vi "FGV_PROXY_connection_references.vi"(6 "station":T1, 7 "options":T2, 8 "error_in":errorcluster, 11 "reference_in":refnum<k5>) -> (0 "error_out":errorcluster, 1 "killed?":bool, 2 "connection_ID_out":refnum<k5>, 3 "listener_ID_out":refnum<k5>)   [LabVIEW 2020]
uses:
  FGV_PROXY_connection_references.ctl
  STATION/station.ctl
  main_ini/FGV_PROXY_config_info.ctl
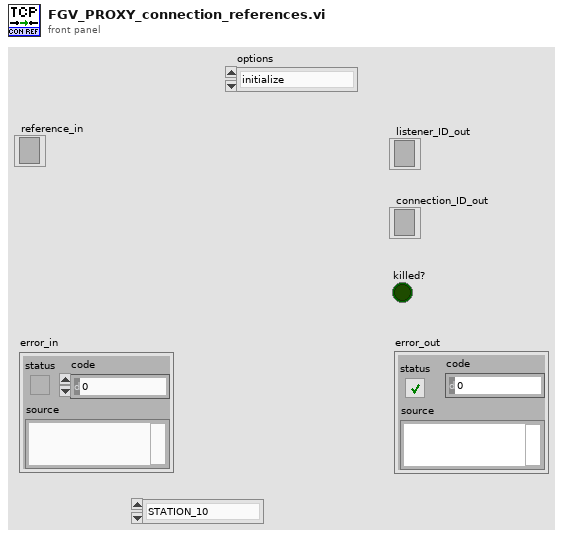
[diagram p1: front panel]
types:
  T1 = typedef "station.ctl" = enum16{"STATION_10", "STATION_20", "STATION_30", "STATION_40", "STATION_50", "STATION_60", "STATION_70", "STATION_80", "STATION_90", "STATION_100", "STATION_110", "STATION_120", "STATION_165", "MAIN"}
  T2 = typedef "FGV_PROXY_connection_references.ctl" = enum16{"initialize", "set_listener_ID", "set_connection_ID", "get", "KILL_ALL_CONNECTIONS", "killed?"}
  T3 = typedef "FGV_PROXY_config_info.ctl" = enum16{"initialize", "set", "get"}
  T4 = typedef "PROXY_all_config_info.ctl" = cluster{"main_ini_file":T5, "SQL Password":string, "queue_refnums":T6, "number_of_stations":i32}
  T5 = typedef "PROXY_main_ini_file.ctl" = cluster{"SQL Driver":string, "SQL Server":string, "SQL Database":string, "SQL UID":string, "Reference table":string, "Reference history":string, "Archivisation CFG table":string, "Archivisation CFG history":string, "User table":string, "User history":string, "default language":string, "REF CHG listener IP":string, "REF CHG listener port":u16, "ST 10 name":string, "ST 10 listener IP":string, "ST 10 listener port":u16, "ST 20 name":string, "ST 20 listener IP":string, "ST 20 listener port":u16, "ST 30 name":string, "ST 30 listener IP":string, "ST 30 listener port":u16, "ST 40 name":string, "ST 40 listener IP":string, "ST 40 listener port":u16, "ST 50 name":string, "ST 50 listener IP":string, "ST 50 listener port":u16, "ST 60 name":string, "ST 60 listener IP":string, "ST 60 listener port":u16, "ST 70 name":string, "ST 70 listener IP":string, "ST 70 listener port":u16, "ST 80 name":string, "ST 80 listener IP":string, "ST 80 listener port":u16, "ST 90 name":string, "ST 90 listener IP":string, "ST 90 listener port":u16, "ST 100 name":string, "ST 100 listener IP":string, "ST 100 listener port":u16, "ST 110 name":string, "ST 110 listener IP":string, "ST 110 listener port":u16, "ST 120 name":string, "ST 120 listener IP":string, "ST 120 listener port":u16, "ST 165 name":string, "ST 165 listener IP":string, "ST 165 listener port":u16}
  T6 = typedef "PROXY_queue_refnums.ctl" = cluster{"ST_10_queue":refnum<queue>, "ST_20_queue":refnum<queue>, "ST_30_queue":refnum<queue>, "ST_40_queue":refnum<queue>, "ST_50_queue":refnum<queue>, "ST_60_queue":refnum<queue>, "ST_70_queue":refnum<queue>, "ST_80_queue":refnum<queue>, "ST_90_queue":refnum<queue>, "ST_100_queue":refnum<queue>, "ST_110_queue":refnum<queue>, "ST_120_queue":refnum<queue>, "ST_165_queue":refnum<queue>}
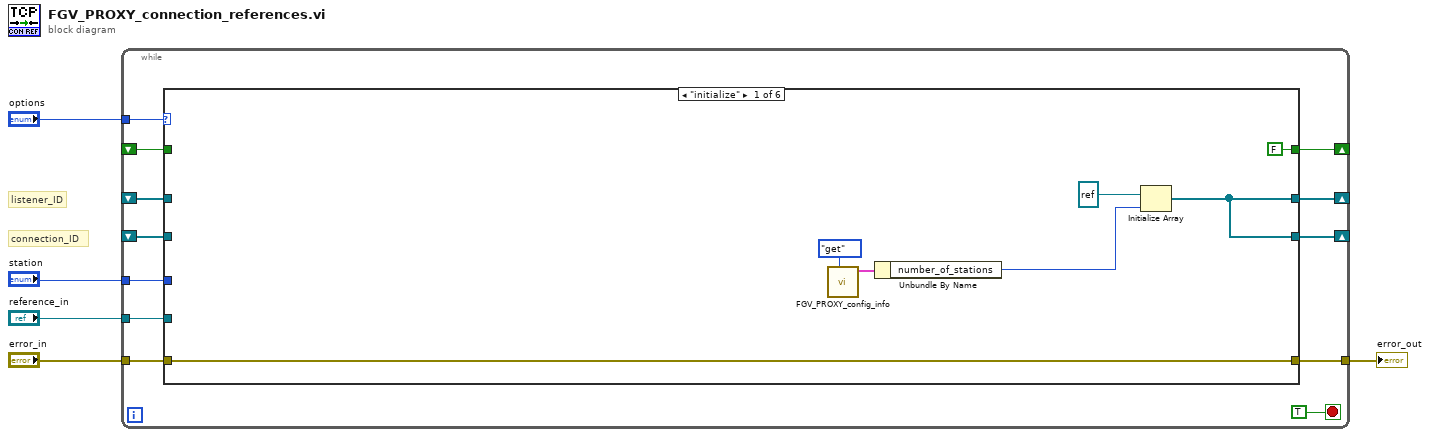
[diagram p0: block diagram]
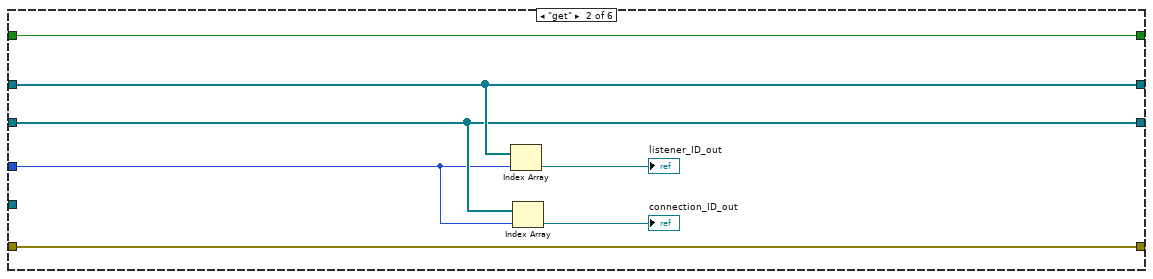
[diagram p2: hidden frame]
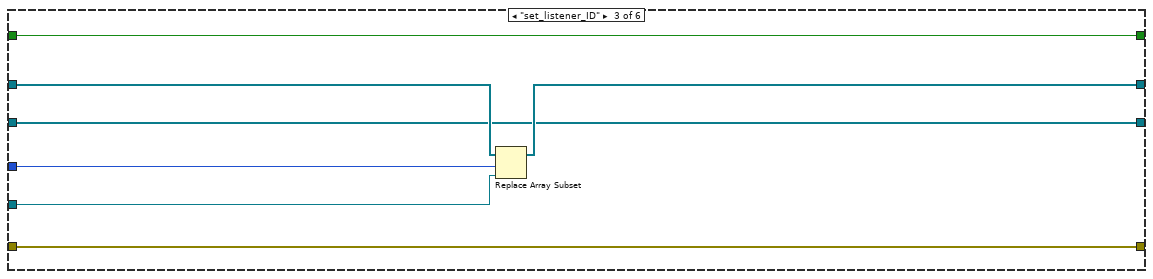
[diagram p3: hidden frame]
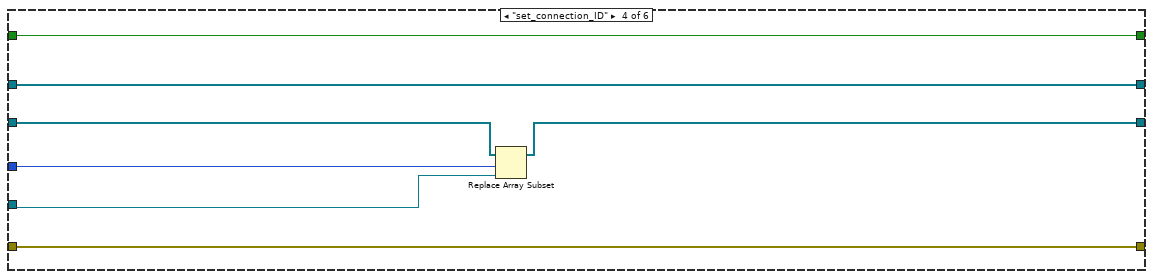
[diagram p4: hidden frame]
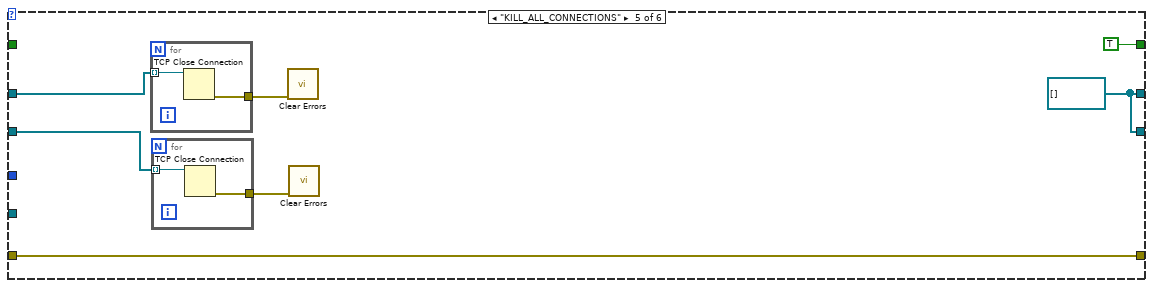
[diagram p5: hidden frame]
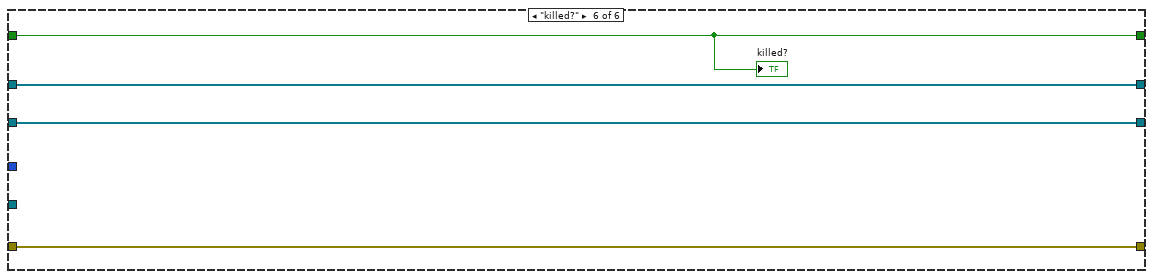
[diagram p6: hidden frame]
diagram:
  # "connection_ID"
  # "listener_ID"
  n1 = while {
    tunnel: "options" -> [w16]
    tunnel: [w15] -> w5
    tunnel: "error_in" -> [w14]
    shift-right: [w13] -> _
    shift-left: _ -> [w10]
    tunnel: "station" -> [w12]
    tunnel: "reference_in" -> [w11]
    shift-right: [w9] -> _
    shift-left: _ -> [w8]
    shift-right: [w7] -> _
    shift-left: _ -> [w6]
    stop <- TRUE stop-if-true
    n2 = case shown="\"initialize\"" w16 {
      tunnel: [w24 w31 w35 w44 w52 w58] -> w15
      tunnel: w14 -> [w24 w31 w35 w44 w52 w58]
      tunnel: [w22 w30 w36 w40 w51 w60] -> w13
      tunnel: w10 -> [_ w30 w38 w40 w50 w60]
      tunnel: w12 -> [_ w27 w37 w45 _ _]
      tunnel: w11 -> [_ _ w34 w41 _ _]
      tunnel: [w22 w28 w33 w43 w51 w59] -> w9
      tunnel: w8 -> [_ w28 w33 w42 w47 w59]
      tunnel: [FALSE w25 w32 w39 TRUE w57] -> w7
      tunnel: w6 -> [_ w25 w32 w39 _ w57]
      frame "initialize" {
        n3 = call "FGV_PROXY_config_info.vi"("options"=FGV_PROXY_config_info."get") -> ("all_config_info_out"=w19:T4)  [unwired: 9 in, 1 out]
        n4 = Unbundle By Name(w19) -> ("number_of_stations"=w18:i32)
        n5 = Initialize Array(refnum<k5> refnum ("connection ID"), w18) -> (w22:refnum<k5>[])
      }
      frame "get" {
        n6 = Index Array(array=w30, index=w27) -> (element=→"listener_ID_out":refnum<k5>)
        n7 = Index Array(array=w28, index=w27) -> (element=→"connection_ID_out":refnum<k5>)
      }
      frame "set_listener_ID" {
        n8 = Replace Array Subset(array=w38, new element=w34, index=w37) -> (w36:refnum<k5>[])
      }
      frame "set_connection_ID" {
        n9 = Replace Array Subset(array=w42, new element=w41, index=w45) -> (w43:refnum<k5>[])
      }
      frame "KILL_ALL_CONNECTIONS" {
        w51 = refnum<k5>[] []
        n10 = for {
          tunnel: w50 -> [w56] mode=indexing
          tunnel: [w55] -> w49
          n11 = TCP Close Connection(connection ID=w56) -> (error out=w55:errorcluster)  [unwired: 2 in, 1 out]
        }
        n12 = for {
          tunnel: w47 -> [w54] mode=indexing
          tunnel: [w53] -> w48
          n13 = TCP Close Connection(connection ID=w54) -> (error out=w53:errorcluster)  [unwired: 2 in, 1 out]
        }
        n14 = call <vilib>:"Clear Errors.vi"("error in (no error)"=w49) -> ()  [unwired: 5 in, 2 out]
        n15 = call <vilib>:"Clear Errors.vi"("error in (no error)"=w48) -> ()  [unwired: 5 in, 2 out]
      }
      frame "killed?" {
        "killed?" <- w57
      }
    }
  }
  "error_out" <- w5
